vi "Parse-Sort-Split.vi"(7 "Include High Priority?":bool, 8 "Error In":errorcluster, 11 "SR List In":T1[](array[typedef])) -> (0 "Error Out":errorcluster, 2 "Unassigned SR List":T1[](array[typedef]), 3 "Assigned SR List":T1[](array[typedef]))   [LabVIEW 2017, in "Client.lvlib"]
uses:
  Client.lvlib
  ParserSorter/SR Data.ctl
  ParserSorter/AE Group.ctl
  ParserSorter/SR Status.ctl
  ParserSorter/SR Level.ctl
  ParserSorter/SR Type.ctl
  ParserSorter/ParserSorter.lvlib
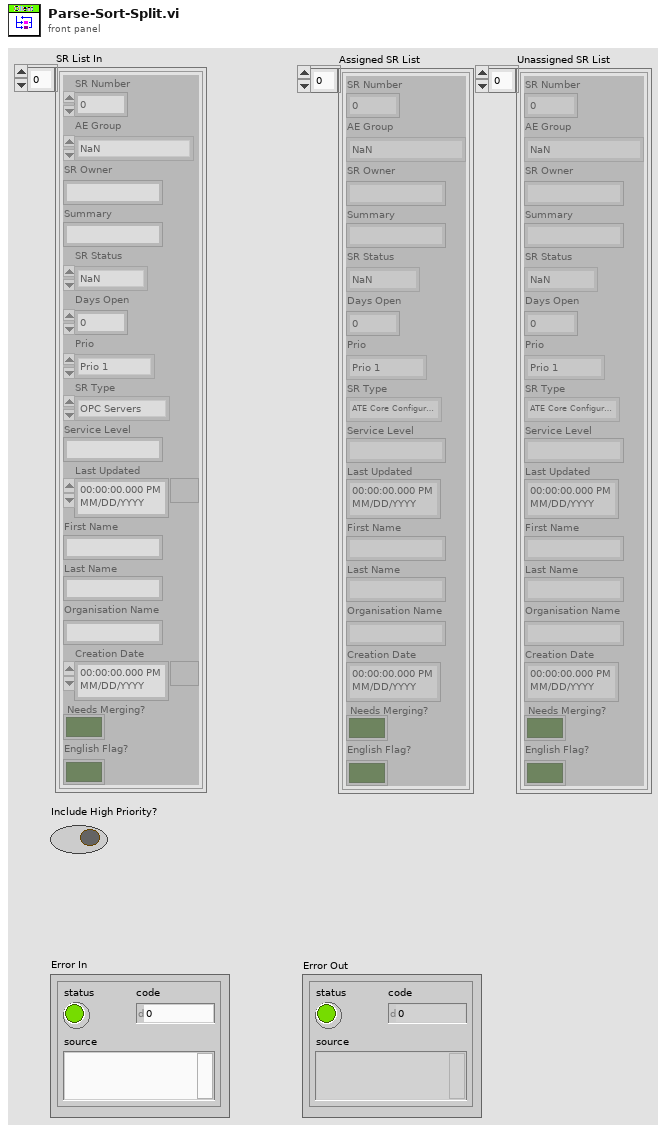
[diagram p1: front panel]
types:
  T1 = typedef "Client.lvlib/ParserSorter.lvlib/SR Data.ctl" = cluster{"SR Number":i64, "AE Group":T2, "SR Owner":string, "Summary":string, "SR Status":T3, "Days Open":dbl, "Prio":T4, "SR Type":T5, "Service Level":string, "Last Updated":timestamp, "First Name":string, "Last Name":string, "Organisation Name":string, "Creation Date":timestamp, "Needs Merging?":bool, "English Flag?":bool}
  T2 = typedef "Client.lvlib/ParserSorter.lvlib/AE Group.ctl" = enum32{"NaN", "AE-Germany", "AE-Poland", "AE-Switzerland", "AE-Czech Republic", "AE-Hungary", "AE-Romania", "AE-Slovakia", "AE-Slovenia"}
  T3 = typedef "Client.lvlib/ParserSorter.lvlib/SR Status.ctl" = enum32{"NaN", "Caller Abandoned", "Created in Error", "Declined to Purchase Support", "Expired", "Forum Resolved AE", "Forum Resolved Customer", "IN WORK", "IN WORK Collab with AES", "IN WORK Collab with PSE", "IN WORK Collab with SE", "IN WORK Escalation", "IN WORK Customer Added Note", "Open", "Potentially Resolved", "POC Resolved", "Resolved", "RMA Waiting on Customer", "RMA Open", "RMA In Progress", "RMA Closed - DOA", "RMA Closed", "RMA Approved for Return", "Project Complete", "Presumed Resolved", "IN WORK Wait on Customer"}
  T4 = typedef "Client.lvlib/ParserSorter.lvlib/SR Level.ctl" = enum16{"Prio 1", "Prio 2", "Prio 3", "Prio 4"}
  T5 = typedef "Client.lvlib/ParserSorter.lvlib/SR Type.ctl" = enum32{"NaN", "ATE Core Configurations (BYOATE)", "Activation", "BioBench", "CAN", "CM C Series", "Calibration", "Consulting Services", "CounterTimer", "DAQExpress", "DASYLab", "DIAdem", "DMM", "DSA HW", "Digital_IO", "FIRST (NIC Only)", "FieldBus", "FieldPoint", "Functional Savety", "GATI", "GPIB", "HMI and Industrial PCs", "HiQ", "HighSpeedDigital_IO", "IMAQ", "IOTech Vibration", "Industrial Communications", "InsightCM", "LV", "LV CD&Sim", "LV Comms", "LV Controls Add-Ons", "LV Embedded", "LV MathScript RT", "LV NXG", "LV NXT", "LVDSC", "LVFPGA", "LVPDA and LV Touch Panel", "LVRT", "LabWindows_CVI", "Lookout", "MATRIXx", "MStudioDotNet", "MStudioVisualBasic", "MStudioVisualC", "Measure (Legacy)", "Motion", "MultifunctionDAQ", "Multimedia Test HW/SW", "Multisim (EWB)", "NI Update Service", "OPC Servers", "Optical (OSI)", "PXI Controllers, Chassis, MXI", "PXI Timing and Sync", "Power Supplies and SMUs", "Powertrain Controls", "RAID", "RF", "RF Software", "RIO", "SC Express", "SCC", "SCXI", "SPEEDY-33 (Hyperception)", "STS", "ScopeDigitizers", "Serial", "Signal Sources", "SignalCondOther", "SignalExpress", "Software Defined Intruments", "Sound and Vibration SW", "Switch Executive", "Switches", "TestStand", "USRP", "Ultiboard (EWB)", "VBench", "VI Logger", "VXI_MXI", "VeriStand", "VisionSW", "VolumeLicenseMgr", "WSN", "Web UI Builder", "myRIO"}
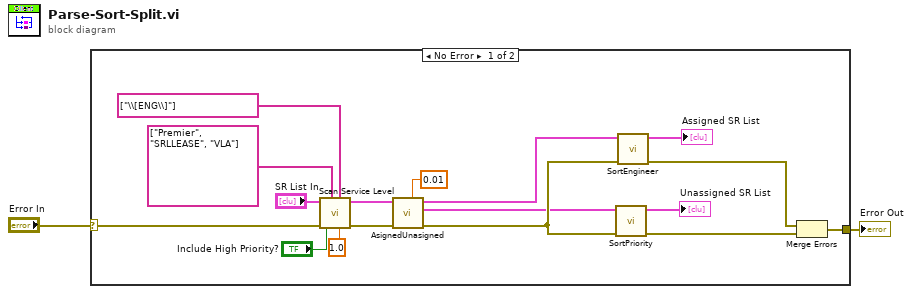
[diagram p0: block diagram]
diagram:
  n1 = case shown="No Error" "Error In" {
    selector: "Error In" -> [w16 w20]
    tunnel: [w8 w20] -> w1
    frame No Error {
      n2 = call "Scan Service Level.vi"("Days Open Prio Threshold"=1.0, "English Tags"=string[] ["\\[ENG\\]"], "Include High Priority?"="Include High Priority?", "Premier Levels Keywords"=string[] ["Premier", "SRLLEASE", "VLA"], "error in (no error)"=w16, "Array in"="SR List In") -> ("error out"=w15:errorcluster, "Array out"=w14:T1[])  [unwired: 4 in]
      n3 = call "AsignedUnasigned.vi"("Days Open Phone Treshhold"=0.01, "error in (no error)"=w15, "All SR In"=w14) -> ("error out"=w12:errorcluster, "Unassigned"=w10:T1[], "Assigned Out"=w11:T1[])  [unwired: 6 in]
      n4 = call "SortPriority.vi"("error in (no error)"=w12, "Array in"=w10) -> ("error out"=w6:errorcluster, "Array out"=→"Unassigned SR List":T1[])  [unwired: 8 in]
      n5 = call "SortEngineer.vi"("error in (no error)"=w12, "Array in"=w11) -> ("error out"=w7:errorcluster, "Array out"=→"Assigned SR List":T1[])  [unwired: 8 in]
      n6 = Merge Errors(w7, w6) -> (w8:errorcluster)
    }
    frame Error {
    }
  }
  "Error Out" <- w1
